vi "getPaths.vi"(8 "error in (no error)":errorcluster, 11 "reference in":refnum<class "File Controller.lvclass">) -> (0 "error out":errorcluster, 2 "paths":T1, 3 "reference out":refnum<class "File Controller.lvclass">)   [LabVIEW 2016, in "File Controller.lvclass"]
uses:
  File Controller.lvclass
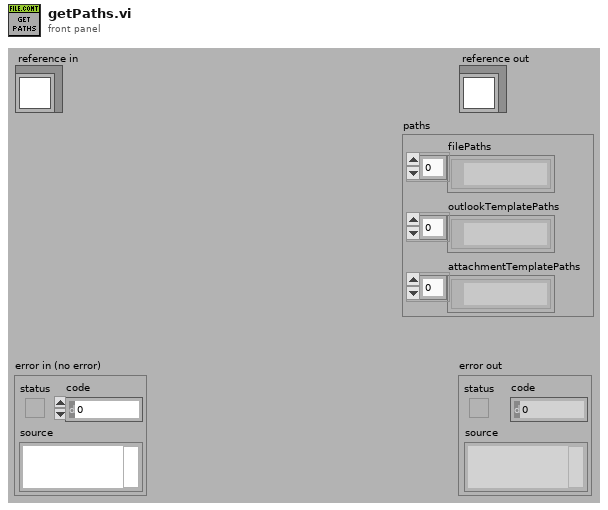
[diagram p1: front panel]
types:
  T1 = cluster{"filePaths":path[], "outlookTemplatePaths":path[], "attachmentTemplatePaths":path[]}
  T2 = typedef "File Controller.lvclass/ObjectAttributesRef.ctl" = refnum<data-value>
  T3 = typedef "File Controller.lvclass/ObjectAttributes.ctl" = cluster{"MyAttribute":dbl, "excelFile_refs":refnum<class "excelFile.lvclass">[], "filePaths":path[], "outlookTemplatePaths":path[], "attachmentTemplatePaths":path[], "configFilePath":path, "not_setting":bool[], "python_ref":refnum<class "python.lvclass">, "TSR":cluster{"number":string, "TSR_path":path, "service_path":path, "email_to":string}}
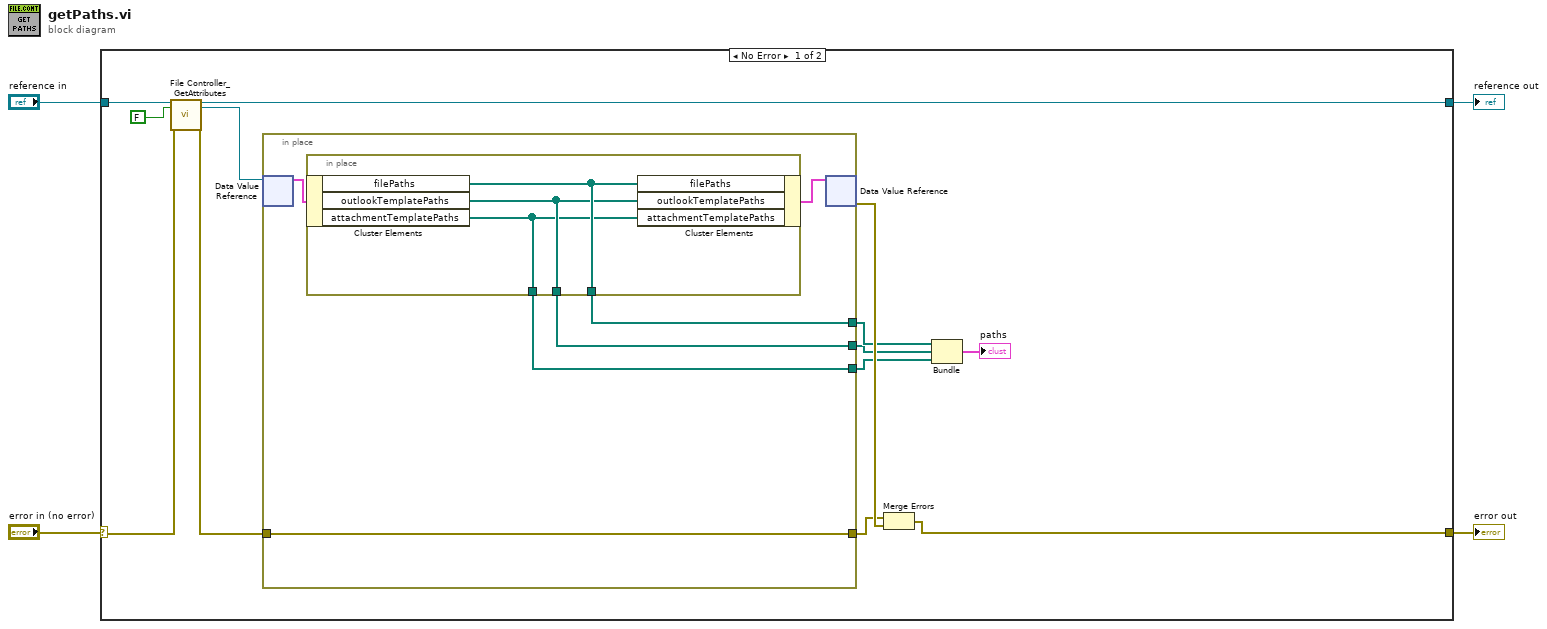
[diagram p0: block diagram]
diagram:
  n1 = case shown="No Error" "error in (no error)" {
    selector: "error in (no error)" -> [w12 w28]
    tunnel: [w17 w28] -> w3
    tunnel: [w10 w27] -> w1
    tunnel: "reference in" -> [w14 w27]
    frame No Error {
      n2 = call "File Controller_GetAttributes.vi"("reference in"=w14, "return data? (T)"=FALSE, "error in (no error)"=w12) -> ("reference out"=w10:refnum<class "File Controller.lvclass">, "attributes ref"=w9:T2, "error out"=w11:errorcluster)  [unwired: 13 in, 1 out]
      n3 = in-place {
        in-place-border: w11 -> [w21]
        in-place-border: [w21] -> w15
        in-place-border: [w20] -> w8
        in-place-border: [w19] -> w7
        in-place-border: [w18] -> w6
        n4 = in-place-dvr #1(w9) -> (w22:T3)  [unwired: 1 out]
        n5 = in-place {
          in-place-border: [w26] -> w20
          in-place-border: [w25] -> w19
          in-place-border: [w24] -> w18
          n6 = in-place-cluster #2(w22) -> ("filePaths"=w26:path[], "outlookTemplatePaths"=w25:path[], "attachmentTemplatePaths"=w24:path[])
          n7 = in-place-cluster #2("filePaths"=w26, "outlookTemplatePaths"=w25, "attachmentTemplatePaths"=w24) -> (w23:T3)
        }
        n8 = in-place-dvr #1(w23) -> (w16:errorcluster)  [unwired: 1 out]
      }
      n9 = Merge Errors(w15, w16) -> (w17:errorcluster)
      n10 = Bundle("filePaths"=w8, "outlookTemplatePaths"=w7, "attachmentTemplatePaths"=w6) -> (→"paths":T1)  [unwired: 1 in]
    }
    frame Error {
    }
  }
  "error out" <- w3
  "reference out" <- w1
